vi "SaveChildClassValues.vi"(8 "error in (no error)":errorcluster caption="entrée d'erreur (pas d'erreur)", 11 "MultiHarp150 en entrée":refnum<class "MultiHarp150.lvclass">) -> (0 "error out":errorcluster caption="sortie d'erreur", 3 "MultiHarp150 en sortie":refnum<class "MultiHarp150.lvclass">)   [LabVIEW 2019, in "MultiHarp150.lvclass"]
uses:
  MultiHarp150.lvclass
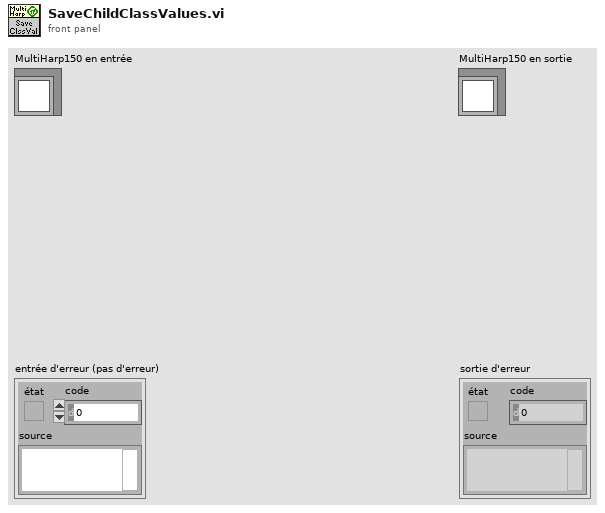
[diagram p1: front panel]
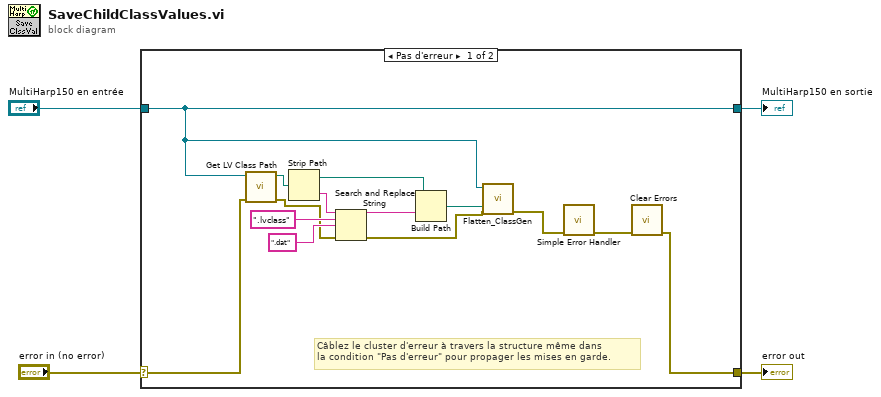
[diagram p0: block diagram]
diagram:
  n1 = case shown="Pas d'erreur" "error in (no error)" {
    selector: "error in (no error)" -> [w10 w20]
    tunnel: [w9 w20] -> w3
    tunnel: [w5 w19] -> w1
    tunnel: "MultiHarp150 en entrée" -> [w5 w19]
    frame No Error {
      # "Câblez le cluster d'erreur à travers la structure même dans\nla condition \"Pas d'erreur\" pour propager les mises en garde."
      n2 = call <vilib>:"Get LV Class Path.vi"("error in (no error)"=w10, "object"=w5) -> ("error out"=w13:errorcluster, "class path"=w18:path)  [unwired: 8 in]
      n3 = Strip Path(path=w18) -> (stripped path=w17:path, name=w16:string)
      n4 = Search and Replace String(input string=w16, search string=".lvclass" ("chaîne recherchée"), replace string=".dat" ("chaîne de remplacement (\"\")"), error in=w13) -> (result string=w12:string, error out=w7:errorcluster)  [unwired: 4 in, 2 out]
      n5 = Build Path(base path=w17, name or relative path=w12) -> (appended path=w8:path)
      n6 = call <userlib>:"Flatten_ClassGen.vi"("error in (no error)"=w7, "XML File Path"=w8, "Objet LabVIEW"=w5) -> ("error out"=w6:errorcluster)  [unwired: 6 in, 2 out]
      n7 = call <vilib>:"Simple Error Handler.vi"("error in (no error)"=w6) -> ("error out"=w11:errorcluster)  [unwired: 4 in, 4 out]
      n8 = call <vilib>:"Clear Errors.vi"("error in (no error)"=w11) -> ("error out"=w9:errorcluster)  [unwired: 5 in, 1 out]
    }
    frame Error {
    }
  }
  "error out" <- w3
  "MultiHarp150 en sortie" <- w1
